vi "readEmcy.vi"(8 "error in (no error)":errorcluster, 10 "emergency object in":refnum<k20>, 11 "MotorController in":refnum<class "MotorController.lvclass">) -> (0 "error out":errorcluster, 1 "emergency message":T1, 2 "emergency object out":refnum<k20>, 3 "MotorController out":refnum<class "MotorController.lvclass">, 5 "isNewMessage":bool)   [LabVIEW 2018, in "MotorController.lvclass"]
uses:
  MotorController.lvclass
  <vilib>/CANopenLib/CANOPEN.llb/CANopen Emergency Read.vi
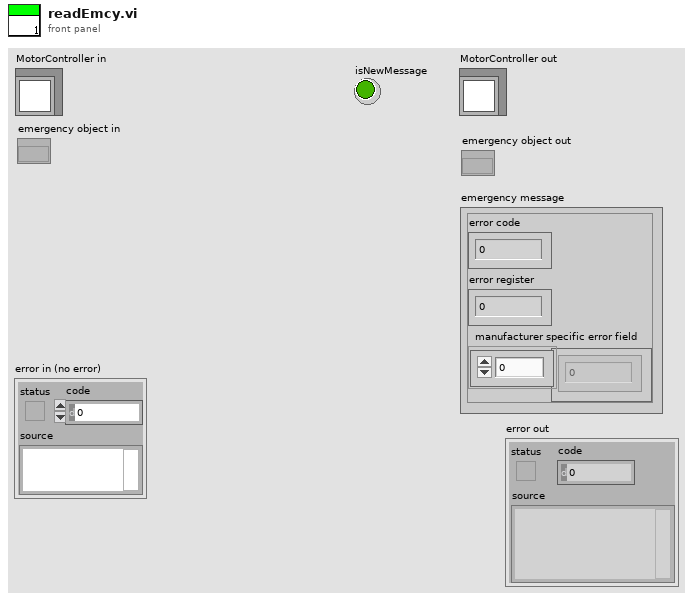
[diagram p1: front panel]
types:
  T1 = cluster{"error code":dbl, "error register":dbl, "manufacturer specific error field":dbl[]}
  T2 = cluster{"error code":u16, "error register":u8, "manufacturer specific error field":u8[]}
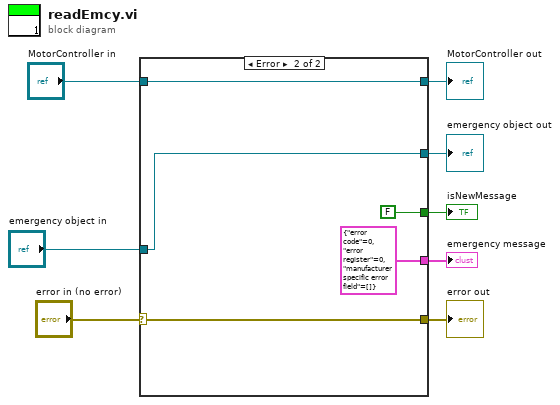
[diagram p0: block diagram]
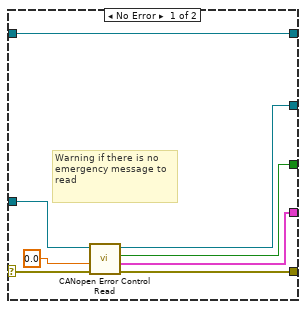
[diagram p2: hidden frame]
diagram:
  n1 = case shown="Error" "error in (no error)" {
    selector: "error in (no error)" -> [w13 w21]
    tunnel: [w9 w21] -> w7
    tunnel: [w11 w20] -> w5
    tunnel: "MotorController in" -> [w11 w20]
    tunnel: [w15 FALSE ("new message?")] -> w4
    tunnel: [w14 T2 {"error code"=0, "error register"=0, "manufacturer specific error field"=[]} ("emergency message")] -> w3
    tunnel: "emergency object in" -> [w12 w17]
    tunnel: [w10 w17] -> w1
    frame No Error {
      # "Warning if there is no emergency message to read"
      n2 = call-poly <vilib>:"CANopen Error Control Read.vi"("error in (no error)"=w13, "timeout (0s)"=0.0, "emergency object in"=w12) -> ("error out"=w9:errorcluster, "emergency message"=w14:T2, "new message?"=w15:bool, "emergency object out"=w10:refnum<k20>)  [unwired: 4 in, 1 out]
    }
    frame Error {
    }
  }
  "error out" <- w7
  "MotorController out" <- w5
  "emergency message" <- w3
  "isNewMessage" <- w4
  "emergency object out" <- w1
